vi "Load Config_File Filter.vi"(8 "error in (no error)":errorcluster, 11 "Refnum in":T2) -> (0 "error out":errorcluster, 2 "File Filter":T1, 3 "Refnum out":T2)   [LabVIEW 2019, in "AutoMenuCreator.lvlib"]
uses:
  AutoMenuCreator.lvlib
  <vilib>/Utility/config.llb/Config Data RefNum.ctl
  Ctl/Ctl_Config_File Filter.ctl
  <vilib>/Utility/config.llb/NI_LVConfig.lvlib
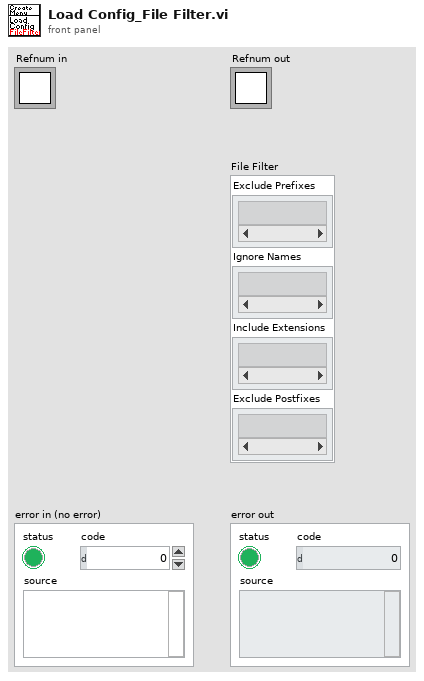
[diagram p1: front panel]
types:
  T1 = typedef "AutoMenuCreator.lvlib/Ctl_Config_File Filter.ctl" = cluster{"Exclude Prefixes":string[], "Ignore Names":string[], "Include Extensions":string[], "Exclude Postfixes":string[]}
  T2 = typedef "NI_LVConfig.lvlib/Config Data RefNum.ctl" = refnum<k1>
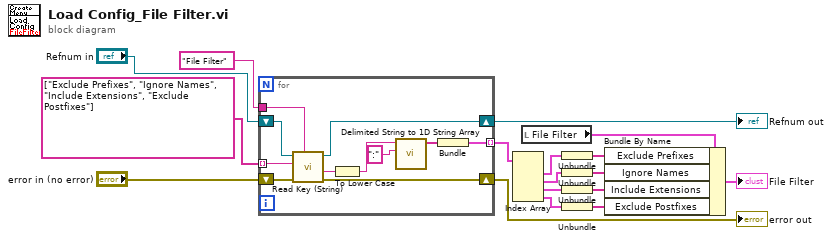
[diagram p0: block diagram]
diagram:
  n1 = for {
    tunnel: "File Filter" ("section") -> [w26]
    shift-right: [w25] -> w13
    shift-left: "Refnum in" -> [w27]
    shift-right: [w24] -> w12
    shift-left: "error in (no error)" -> [w28]
    tunnel: string[] ["Exclude Prefixes", "Ignore Names", "Include Extensions", "Exclude Postfixes"] ("key") -> [w23] mode=indexing
    tunnel: [w19] -> w11 mode=indexing
    n2 = call <vilib>:"Read Key (String).vi"("section"=w26, "error in (no error)"=w28, "key"=w23, "refnum"=w27) -> ("error out"=w24:errorcluster, "value"=w22:string, "refnum out"=w25:T2)  [unwired: 4 in, 1 out]
    n3 = To Lower Case(string=w22) -> (all lower case string=w18:string)
    n4 = call <vilib>:"Delimited String to 1D String Array.vi"("delimiter"=":", "delimited string"=w18) -> ("string array"=w20:string[])  [unwired: 9 in]
    n5 = Bundle("string array"=w20) -> (w19:cluster{"string array":string[]})  [unwired: 1 in]
  }
  "error out" <- w12
  "Refnum out" <- w13
  n6 = Index Array(array=w11) -> (element #1=w10:cluster{"string array":string[]}, element #2=w9:cluster{"string array":string[]}, element #3=w8:cluster{"string array":string[]}, element #4=w1:cluster{"string array":string[]})  [unwired: 4 in]
  n7 = local read "File Filter"() -> (w3:T1)
  n8 = Unbundle(w10) -> ("string array"=w7:string[])
  n9 = Unbundle(w9) -> ("string array"=w6:string[])
  n10 = Unbundle(w8) -> ("string array"=w5:string[])
  n11 = Unbundle(w1) -> ("string array"=w2:string[])
  n12 = Bundle By Name(cluster=w3, "Exclude Prefixes"=w7, "Ignore Names"=w6, "Include Extensions"=w5, "Exclude Postfixes"=w2) -> (→"File Filter":T1)
